vi "Popup.vi"(8 "error in (no error)":errorcluster, 10 "Msg":string, 11 "Test-Client in":refnum<class "Test-Client.lvclass">) -> (0 "error out":errorcluster, 3 "Test-Client out":refnum<class "Test-Client.lvclass">)   [LabVIEW 2020, in "Test-Client.lvlib" / "Test-Client.lvclass"]
uses:
  Test-Client.lvclass
  Test-Client.lvclass/Test-Client.ctl
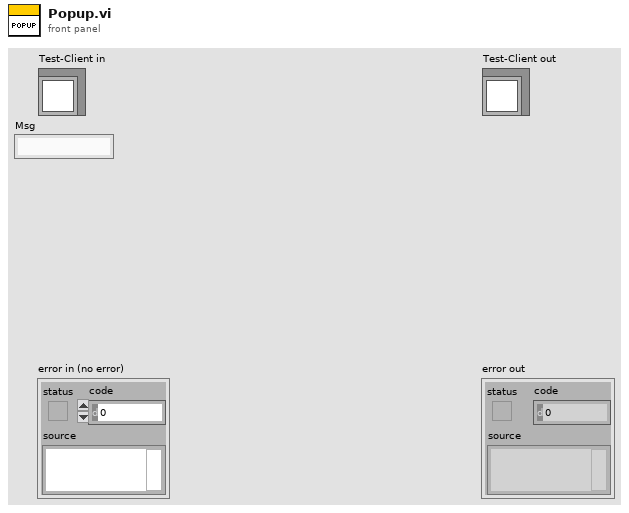
[diagram p1: front panel]
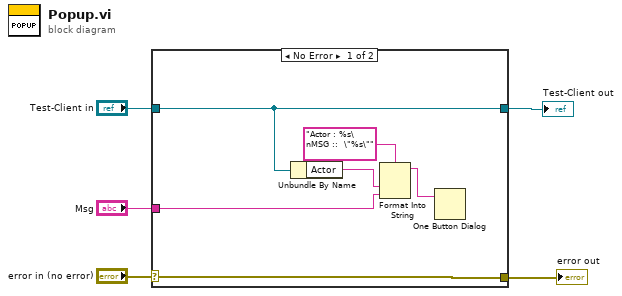
[diagram p0: block diagram]
diagram:
  n1 = case shown="No Error" "error in (no error)" {
    selector: "error in (no error)" -> [w11 w13]
    tunnel: [w11 w13] -> w4
    tunnel: [w10 w12] -> w2
    tunnel: "Test-Client in" -> [w10 w12]
    tunnel: "Msg" -> [w6 _]
    frame No Error {
      n2 = Unbundle By Name(w10) -> ("Actor"=w9:string)
      n3 = Format Into String(format string="Actor : %s\nMSG ::  \"%s\"", w9, w6) -> (resulting string=w8:string)  [unwired: 2 in, 1 out]
      n4 = One Button Dialog(message=w8) -> ()  [unwired: 1 in, 1 out]
    }
    frame Error {
    }
  }
  "error out" <- w4
  "Test-Client out" <- w2
